vi "Create Core.vi"(6 "Custom Config Data":u8[](array[numeric]) format="%.0x", 7 "Direction":T2, 8 "error in (no error)":errorcluster, 9 "Disconnect Behavior":T1, 10 "Name":string, 11 "CIFChannels in":refnum<class "CIFChannels.lvclass">) -> (0 "error out":errorcluster, 1 "Bytes/Msg":u64, 2 "Channel Type":string, 3 "CIFChannels out":refnum<class "CIFChannels.lvclass">, 4 "Messages":u64)   [LabVIEW 2021, in "CIFChannels.lvclass"]
uses:
  CIFChannels.lvclass
  Typedef/Direction.ctl
  Typedef/Disconnect Behavior.ctl
  Typedef/Channel State.ctl
  CIFChannels.lvclass/CIFChannels.ctl
  Accessors/Write Type.vi
  Accessors/Write Channel Class.vi
  Accessors/Write Channel State.vi
  Accessors/Write Direction.vi
  Accessors/Write Tag Disconnect Behavior.vi
  Accessors/Write Name.vi
  Accessors/Write Custom Config Data.vi
  <vilib>/CIF Foundation/CIF Utilities/DataTypes/Unflatten U64.vi
  ChannelCommon/Utilities/Expand FIFO Flags.vi
  ChannelCommon/ChannelCommon.lvlib
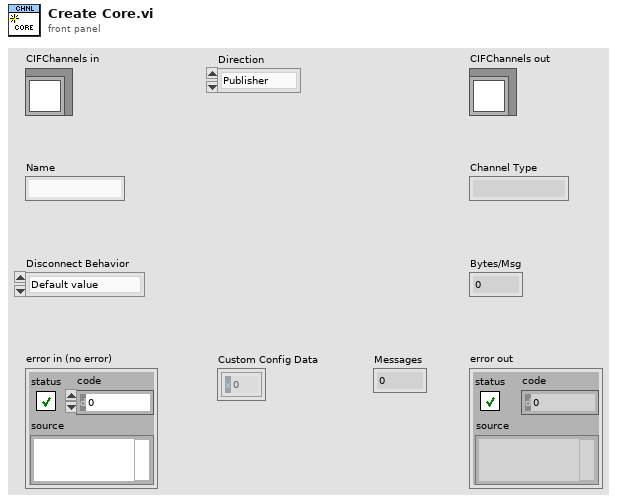
[diagram p1: front panel]
types:
  T1 = typedef "CIFChannels.lvclass/Disconnect Behavior.ctl" = enum16{"Default value", "Last value", "Error with default"}
  T2 = typedef "CIFChannels.lvclass/Direction.ctl" = enum16{"Publisher", "Subscriber"}
  T3 = typedef "CIFChannels.lvclass/Channel State.ctl" = enum16{"Creating", "Disconnected", "Connecting", "Connected", "Destroyed"}
  T4 = typedef "ChannelCommon.lvlib/FIFO Config.ctl" = cluster{"Max Bytes/Msg":u64, "Msg Depth":u64, "Flags":u64}
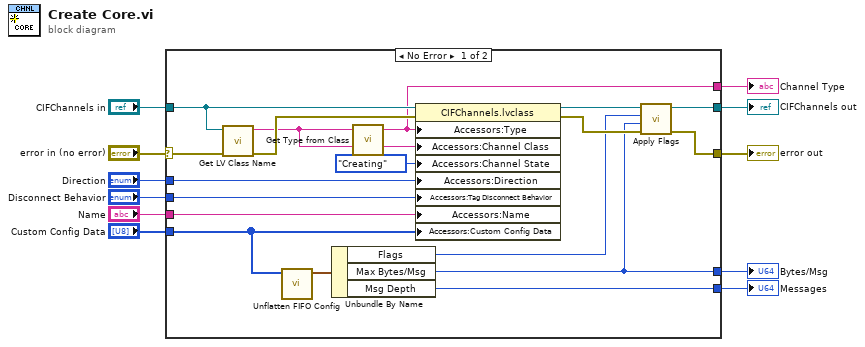
[diagram p0: block diagram]
diagram:
  n1 = case shown="No Error" "error in (no error)" {
    selector: "error in (no error)" -> [w25 w31]
    tunnel: [w16 w31] -> w10
    tunnel: [w15 w30] -> w8
    tunnel: "CIFChannels in" -> [w24 w30]
    tunnel: "Direction" -> [w29 _]
    tunnel: "Name" -> [w28 _]
    tunnel: "Disconnect Behavior" -> [w27 _]
    tunnel: "Custom Config Data" -> [w19 _]
    tunnel: [w22 _] -> w3
    tunnel: [w12 _] -> w2
    tunnel: [w13 _] -> w1
    frame No Error {
      n2 = call <vilib>:"Get LV Class Name.vi"("error in (no error)"=w25, "object"=w24) -> ("error out"=w23:errorcluster, "class name"=w21:string)  [unwired: 8 in]
      n3 = call "Unflatten FIFO Config.vi"("Flattened Data in"=w19) -> ("FIFO Config out"=w20:T4)  [unwired: 9 in, 1 out]
      n4 = Unbundle By Name(w20) -> ("Flags"=w14:u64, "Max Bytes/Msg"=w12:u64, "Msg Depth"=w13:u64)
      n5 = call "Get Type from Class.vi"("Class"=w21) -> ("Channel Type"=w22:string)  [unwired: 4 in]
      n6 = property class="CIFChannels.lvclass"(reference=w24, error in=w23, "Accessors:Type"=w22, "Accessors:Channel Class"=w21, "Accessors:Channel State"=Channel_State."Creating" ("Channel State"), "Accessors:Direction"=w29, "Accessors:Tag Disconnect Behavior"=w27, "Accessors:Name"=w28, "Accessors:Custom Config Data"=w19) -> (reference out=w18:refnum<class "CIFChannels.lvclass">, error out=w17:errorcluster)
      n7 = call "Apply Flags.vi"("error in (no error)"=w17, "Max Bytes/Msg"=w12, "FIFO Flags"=w14, "CIFChannels in"=w18) -> ("error out"=w16:errorcluster, "CIFChannels out"=w15:refnum<class "CIFChannels.lvclass">)  [unwired: 6 in]
    }
    frame Error {
    }
  }
  "error out" <- w10
  "CIFChannels out" <- w8
  "Channel Type" <- w3
  "Bytes/Msg" <- w2
  "Messages" <- w1
